vi "Cycle Fulfill Error.vi"(8 "error in (no error)":errorcluster) -> (0 "error out":errorcluster)   [LabVIEW 2017, in "Unit Tests.lvlib"]
uses:
  Unit Tests.lvlib
  0b9f98d7-229e-4165-85b4-d78c21aa15e7.vi
  e38c4525-3448-4fbc-8db8-7559fd649511.vi
  317b27dd-cc51-42ab-9783-837260827ee9.vi
  Promise Future/Promise/Promise.lvclass
  E:/Promise/Promise Future/Future/Future.lvclass
  Promise Future/Future/Fulfull (Future).vi
  <vilib>/addons/_JKI Toolkits/Caraya/classes/Test/Test.lvclass
  <vilib>/addons/_JKI Toolkits/Caraya/classes/Assert/Assert.lvclass
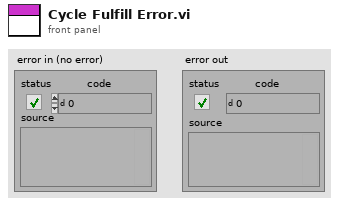
[diagram p1: front panel]
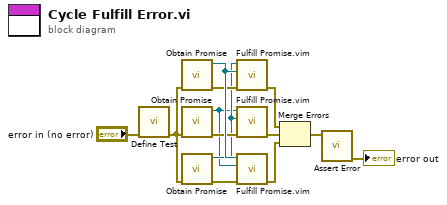
[diagram p0: block diagram]
diagram:
  n1 = call <vilib>:"Define Test.vi"("error in (no error)"="error in (no error)") -> ("error out"=w9:errorcluster)  [unwired: 10 in]
  n2 = call "Obtain Promise.vi"("error in (no error)"=w9) -> ("error out"=w11:errorcluster, "Promise out"=w12:refnum<class "Promise.lvclass">)  [unwired: 8 in, 1 out]
  n3 = call "Obtain Promise.vi"("error in (no error)"=w9) -> ("error out"=w4:errorcluster, "Promise out"=w2:refnum<class "Promise.lvclass">)  [unwired: 8 in, 1 out]
  n4 = call "Obtain Promise.vi"("error in (no error)"=w9) -> ("error out"=w10:errorcluster, "Promise out"=w3:refnum<class "Promise.lvclass">)  [unwired: 8 in, 1 out]
  n5 = call "Fulfill Promise.vim"("error in (no error)"=w11, "Value"=w12, "Promise in"=w3) -> ("error out"=w8:errorcluster)  [unwired: 7 in, 1 out]
  n6 = call "Fulfill Promise.vim"("error in (no error)"=w4, "Value"=w3, "Promise in"=w2) -> ("error out"=w5:errorcluster)  [unwired: 7 in, 1 out]
  n7 = call "Fulfill Promise.vim"("error in (no error)"=w10, "Value"=w2, "Promise in"=w12) -> ("error out"=w7:errorcluster)  [unwired: 7 in, 1 out]
  n8 = Merge Errors(w8, w5, w7) -> (w6:errorcluster)
  n9 = call <vilib>:"Assert Error.vi"("Error?"=w6) -> ("error out"=→"error out":errorcluster)  [unwired: 10 in]
